vi "Teststand Engine Driver.vi"(8 "error in":errorcluster, 11 "Sequence Context In":refnum<k7>) -> (0 "error out":errorcluster)   [LabVIEW 2023, in "HardwareAbstractionLayer_LVOOP.lvlib" / "Teststand.lvclass"]
uses:
  Teststand.lvclass
  Teststand.lvclass/Teststand.ctl
  <vilib>/addons/TestStand/_TSUtility.llb/TestStand - Status Monitor.ctl
  Teststand Steptypes/GlobalVariable/GlobalVariableData.vi
  Teststand Steptypes/LTT_TeststandSteptypes.lvlib
  <vilib>/addons/TestStand/_TSUtility.llb/TestStand - Get Property Value (Boolean).vi
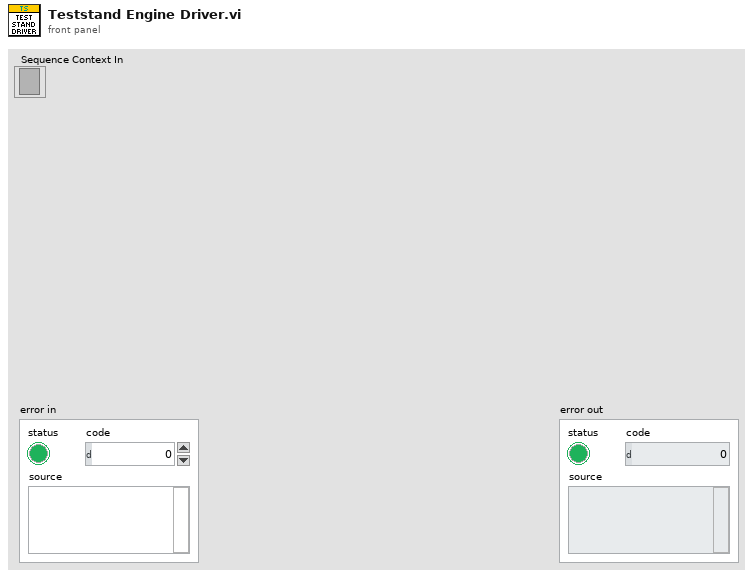
[diagram p1: front panel]
types:
  T1 = typedef "TestStand - Status Monitor.ctl" = cluster{"Sequence Context":refnum<k7>, "Execution":refnum<k7>, "Termination Monitor":refnum<k7>}
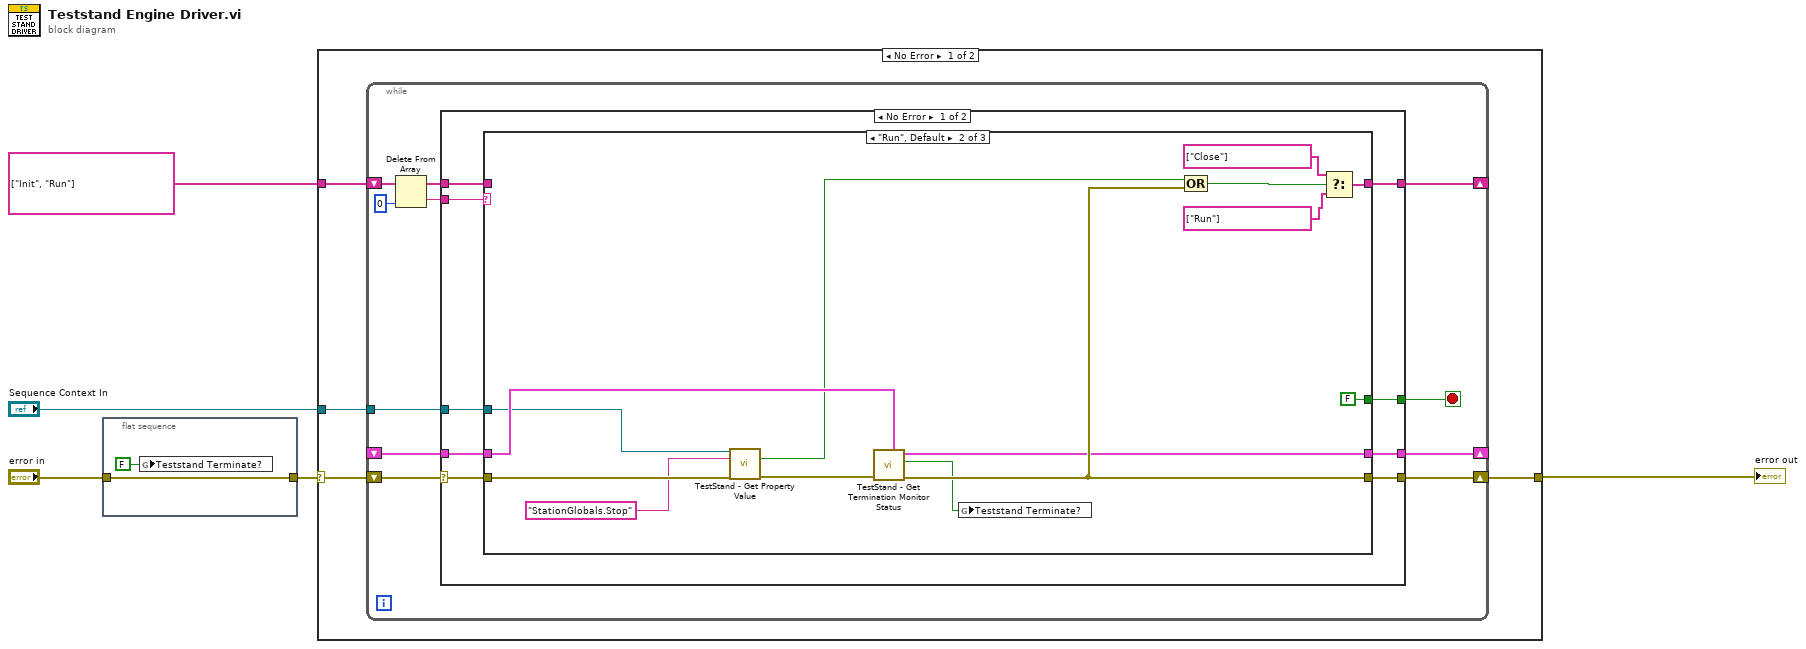
[diagram p0: block diagram]
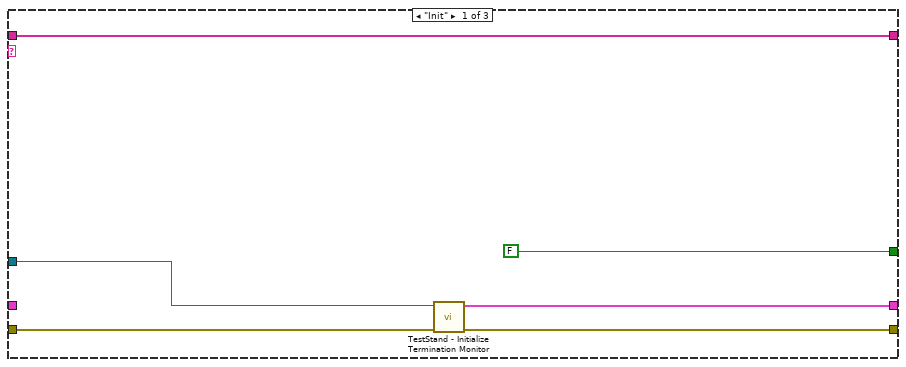
[diagram p2: hidden frame]
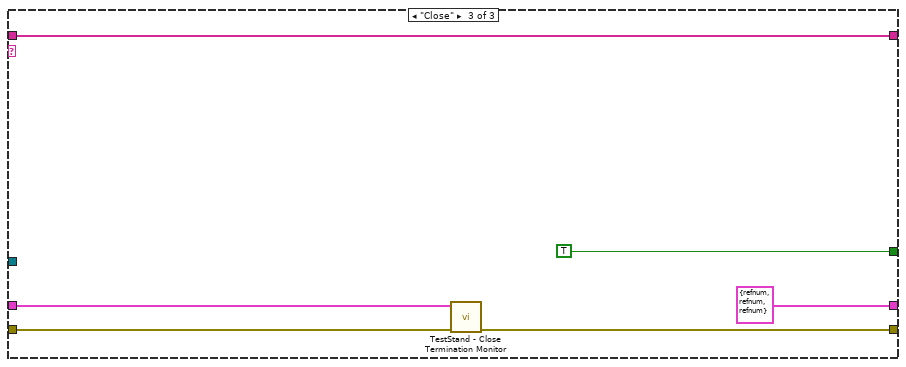
[diagram p3: hidden frame]
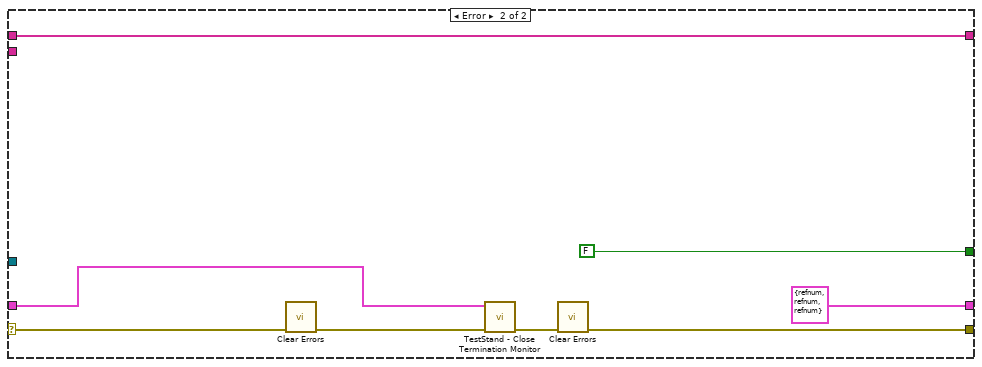
[diagram p4: hidden frame]
diagram:
  n1 = flat-sequence {
    tunnel: "error in" -> [w6]
    tunnel: [w6] -> w1
    frame #0 {
      n2 = global write "GlobalVariableData.vi" "Teststand Terminate?"(FALSE ("Teststand Terminate?")) -> ()
    }
  }
  n3 = case shown="No Error" w1 {
    selector: w1 -> [w11 w66]
    tunnel: [w10 w66] -> w5
    tunnel: string[] ["Init", "Run"] -> [w9 _]
    tunnel: "Sequence Context In" -> [w8 _]
    frame No Error {
      n4 = while {
        shift-right: [w21] -> w10
        shift-left: w11 -> [w22]
        shift-right: [w16] -> _
        shift-left: w9 -> [w20]
        tunnel: w8 -> [w14]
        shift-right: [w13] -> _
        shift-left: _ -> [w12]
        stop <- w15 stop-if-true
        n5 = Delete From Array(array=w20, index=0) -> (deleted portion=w18:string, array with subset deleted=w17:string[])  [unwired: 1 in]
        n6 = case shown="No Error" w22 {
          selector: w22 -> [w28 w62]
          tunnel: [w27 w59] -> w21
          tunnel: w18 -> [w31 _]
          tunnel: w17 -> [w30 w65]
          tunnel: [w29 w65] -> w16
          tunnel: [w26 FALSE] -> w15
          tunnel: w14 -> [w25 _]
          tunnel: [w24 T1 {"Sequence Context"=refnum, "Execution"=refnum, "Termination Monitor"=refnum} ("Status Monitor Out")] -> w13
          tunnel: w12 -> [w23 w58]
          frame No Error {
            n7 = case shown="\"Run\", Default" w31 {
              tunnel: w30 -> [w37 _ w57]
              tunnel: [w37 w49 w57] -> w29
              tunnel: w28 -> [w34 w48 w55]
              tunnel: [w33 w45 w54] -> w27
              tunnel: [FALSE FALSE TRUE] -> w26
              tunnel: w25 -> [w35 w40 _]
              tunnel: [w32 w43 T1 {"Sequence Context"=refnum, "Execution"=refnum, "Termination Monitor"=refnum} ("Status Monitor Out")] -> w24
              tunnel: w23 -> [_ w44 w53]
              frame "Init" {
                n8 = call <vilib>:"TestStand - Initialize Termination Monitor.vi"("error in (no error)"=w34, "Sequence Context In"=w35) -> ("error out"=w33:errorcluster, "Status Monitor Out"=w32:T1)  [unwired: 8 in]
              }
              frame "Run", Default {
                n9 = call-poly <vilib>:"TestStand - Get Property Value.vi"("Sequence Context In"=w40, "Lookup String"="StationGlobals.Stop", "error in (no error)"=w48) -> ("Value"=w38:bool, "error out"=w39:errorcluster)  [unwired: 10 in, 1 out]
                n10 = call <vilib>:"TestStand - Get Termination Monitor Status.vi"("error in (no error)"=w39, "Status Monitor In"=w44) -> ("error out"=w45:errorcluster, "Terminating or Aborting"=w42:bool, "Status Monitor Out"=w43:T1)  [unwired: 7 in]
                n11 = global write "GlobalVariableData.vi" "Teststand Terminate?"(w42) -> ()
                n12 = Compound Arithmetic op=OR(w38, w45) -> (w46:bool)
                n13 = Select(t=string[] ["Close"], s=w46, f=string[] ["Run"]) -> (s? t:f=w49:string[])
              }
              frame "Close" {
                n14 = call <vilib>:"TestStand - Close Termination Monitor.vi"("error in (no error)"=w55, "Status Monitor In"=w53) -> ("error out"=w54:errorcluster)  [unwired: 9 in]
              }
            }
          }
          frame Error {
            n15 = call <vilib>:"Clear Errors.vi"("error in (no error)"=w62) -> ("error out"=w61:errorcluster)  [unwired: 5 in, 1 out]
            n16 = call <vilib>:"TestStand - Close Termination Monitor.vi"("error in (no error)"=w61, "Status Monitor In"=w58) -> ("error out"=w60:errorcluster)  [unwired: 9 in]
            n17 = call <vilib>:"Clear Errors.vi"("error in (no error)"=w60) -> ("error out"=w59:errorcluster)  [unwired: 5 in, 1 out]
          }
        }
      }
    }
    frame Error {
    }
  }
  "error out" <- w5
